vi "Configure test.vi"(6 "Assert VI Path":path, 7 "Existing Queue Elements":string, 8 "error in (no error)":errorcluster, 11 "FP Equal in":refnum<class "FP Equal.lvclass">) -> (0 "error out":errorcluster, 3 "Floating Point out":refnum<class "FP Equal.lvclass">)   [LabVIEW 2018, in "FP Equal.lvclass"]
uses:
  FP Equal.lvclass
  7aea5dfe-153d-450d-a60d-af525a96a8b0.vi
  <vilib>/JDP Science/JSONtext/Find Item.vi
  7aea5dfe-153d-450d-a60d-af525a96a8b0.vi/24006521-a375-4a29-aece-8e626034dc66.vi
  7aea5dfe-153d-450d-a60d-af525a96a8b0.vi/cfab99af-cbc2-48b8-9fbf-106b876cde10.vi
  <vilib>/JDP Science/JSONtext/String Subset.vi
  Test Class String IDs.vi
  <vilib>/JDP Science/JSONtext/Parsing/Parse Full Path or Item Name.vi
  <vilib>/JDP Science/JSONtext/Offset/Find Item Locations by Path.vi
  <vilib>/JDP Science/JSONtext/JSON text to Variant.vi
  <vilib>/JDP Science/JSONtext/Variant to JSON Text.vi
  <vilib>/JDP Science/JSONtext/Set Item.vi
  Floating Point.lvclass
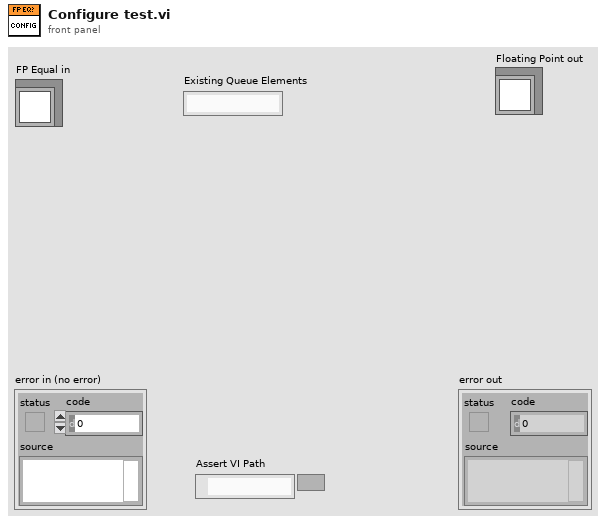
[diagram p1: front panel]
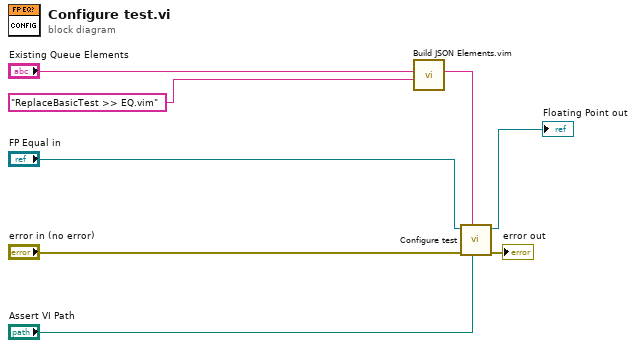
[diagram p0: block diagram]
diagram:
  n1 = call "Build JSON Elements.vim"("Append Element(s)"="ReplaceBasicTest >> EQ.vim", "JSON Elements in ({})"="Existing Queue Elements") -> ("JSON Elements out"=w5:string)  [unwired: 9 in]
  n2 = call-parent "Configure test.vi"("Assert VI Path"="Assert VI Path", "Existing Queue Elements"=w5, "error in (no error)"="error in (no error)", "Floating Point in"="FP Equal in") -> ("error out"=→"error out":errorcluster, "Floating Point out"=→"Floating Point out":refnum<class "FP Equal.lvclass">)  [unwired: 6 in]
